vi "SumArray.vi"(0 "Array":dbl[][](array[numeric])) -> (1 "Sum":dbl, 2 "Average":dbl)   [LabVIEW 2012]
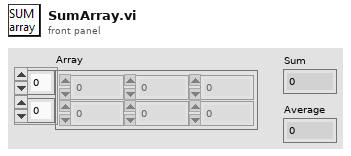
[diagram p1: front panel]
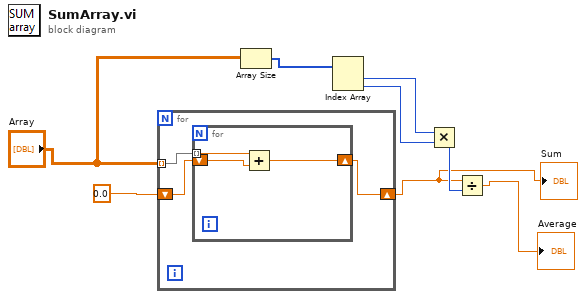
[diagram p0: block diagram]
diagram:
  n1 = for {
    tunnel: "Array" -> [w11] mode=indexing
    shift-right: [w9] -> w1
    shift-left: 0.0 ("y") -> [w10]
    n2 = for {
      tunnel: w11 -> [w14] mode=indexing
      shift-right: [w13] -> w9
      shift-left: w10 -> [w12]
      n3 = Add(x=w14, y=w12) -> (x+y=w13:dbl)
    }
  }
  "Sum" <- w1
  n4 = Array Size(array="Array") -> (size(s)=w5:i32[])
  n5 = Index Array(array=w5) -> (element #1=w4:i32, element #2=w3:i32)  [unwired: 2 in]
  n6 = Multiply(x=w4, y=w3) -> (x*y=w7:i32)
  n7 = Divide(x=w1, y=w7) -> (x/y=→"Average":dbl)
